vi "destroy.vi"(8 "error in":errorcluster, 11 "message connection in":refnum<class "identifying queue.lvclass">) -> (0 "error out":errorcluster)   [LabVIEW 2015, in "identifying queue.lvclass"]
uses:
  identifying queue.lvclass
  identifying queue.lvclass/identifying queue.ctl
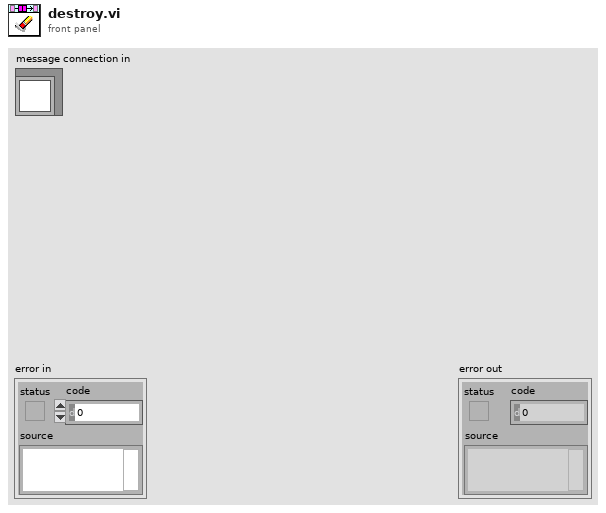
[diagram p1: front panel]
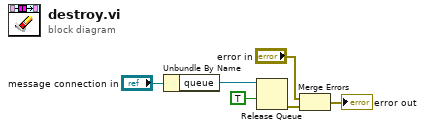
[diagram p0: block diagram]
diagram:
  n1 = Unbundle By Name("message connection in") -> ("queue"=w4:refnum<queue>)
  n2 = Release Queue(queue=w4, force destroy? (F)=TRUE) -> (error out=w6:errorcluster)  [unwired: 1 in, 2 out]
  n3 = Merge Errors("error in", w6) -> (→"error out":errorcluster)
